vi "basic-intro-log.vi"(0 "Recording Location":string="BI Room 146", 1 "Number of trials":string(combo)="200", 2 "Reward Vol. (uL)":dbl=5.0, 3 "Max number of \nconsecutive trials":string(combo)="3", 4 "Min Licks":i32=1 min=1, 5 "ITI upper (s)":dbl=25.0, 6 "ITI lower (s)":dbl=8.0, 8 "Sequence Directory":path=path "C:/Users/SiapasLab/Desktop/git/wheatley", 9 "Punish Time (s)":dbl=25.0, 10 "Data Saving Directory":path=path "\\\\CA1-17\\ld8007/anesthesia/data", 11 "Trial window (ms)":dbl=3000.0, 12 "Animal Name":string="Mouse", 13 "Trial delay (ms)":dbl=2000.0, 14 "Assay Description":string="Two Choice Audio Discrimination", 15 "Max Time (s)":dbl=3600.0, 16 "Tone Pairs":u16(ring) items=["1: CS+ 10000 Hz, CS- 5000 Hz", "2: CS+ 5800 Hz, CS- 5000 Hz", "3: CS+ 5000 Hz, CS- 10000 Hz", "4: CS+ 8000 Hz, CS- 15000 Hz"], 17 "Protocol":u16(ring)=1 items=["Partial Training 1", "Full Training"]) -> (18 "all rows":i64[](array[numeric]), 20 "Cluster":T2, 21 "Cluster 2":T1)   [LabVIEW 2015]
uses:
  <vilib>/Utility/file.llb/Read Delimited Spreadsheet (I64).vi
panel:
  in  "Ring Refnum":refnum<vi>
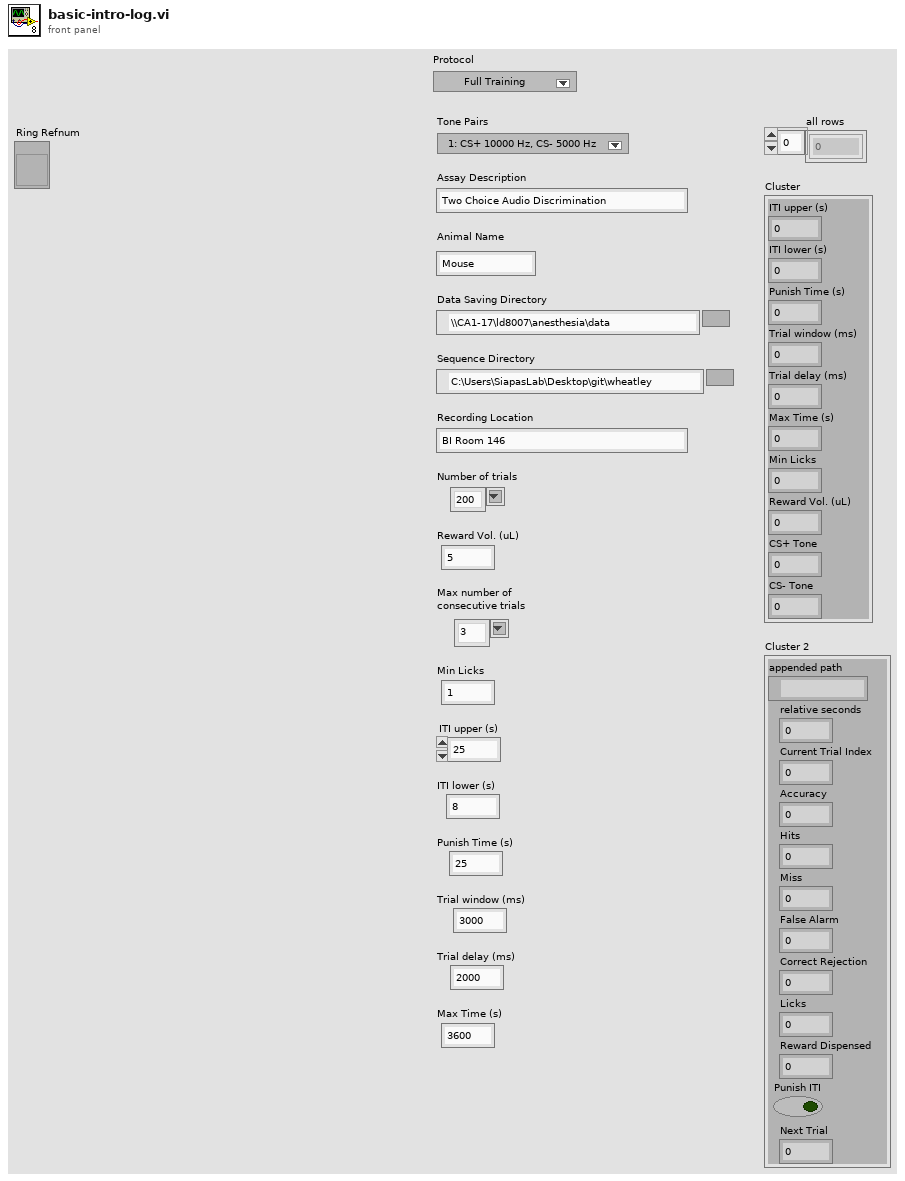
[diagram p1: front panel]
types:
  T1 = cluster{"appended path":path, "relative seconds":dbl, "Current Trial Index":i32, "Accuracy":dbl, "Hits":i32, "Miss":i32, "False Alarm":i32, "Correct Rejection":i32, "Licks":i32, "Reward Dispensed":dbl, "Punish ITI":bool, "Next Trial":i32}
  T2 = cluster{"ITI upper (s)":dbl, "ITI lower (s)":dbl, "Punish Time (s)":dbl, "Trial window (ms)":dbl, "Trial delay (ms)":dbl, "Max Time (s)":dbl, "Min Licks":i32, "Reward Vol. (uL)":dbl, "CS+ Tone":i32, "CS- Tone":i32}
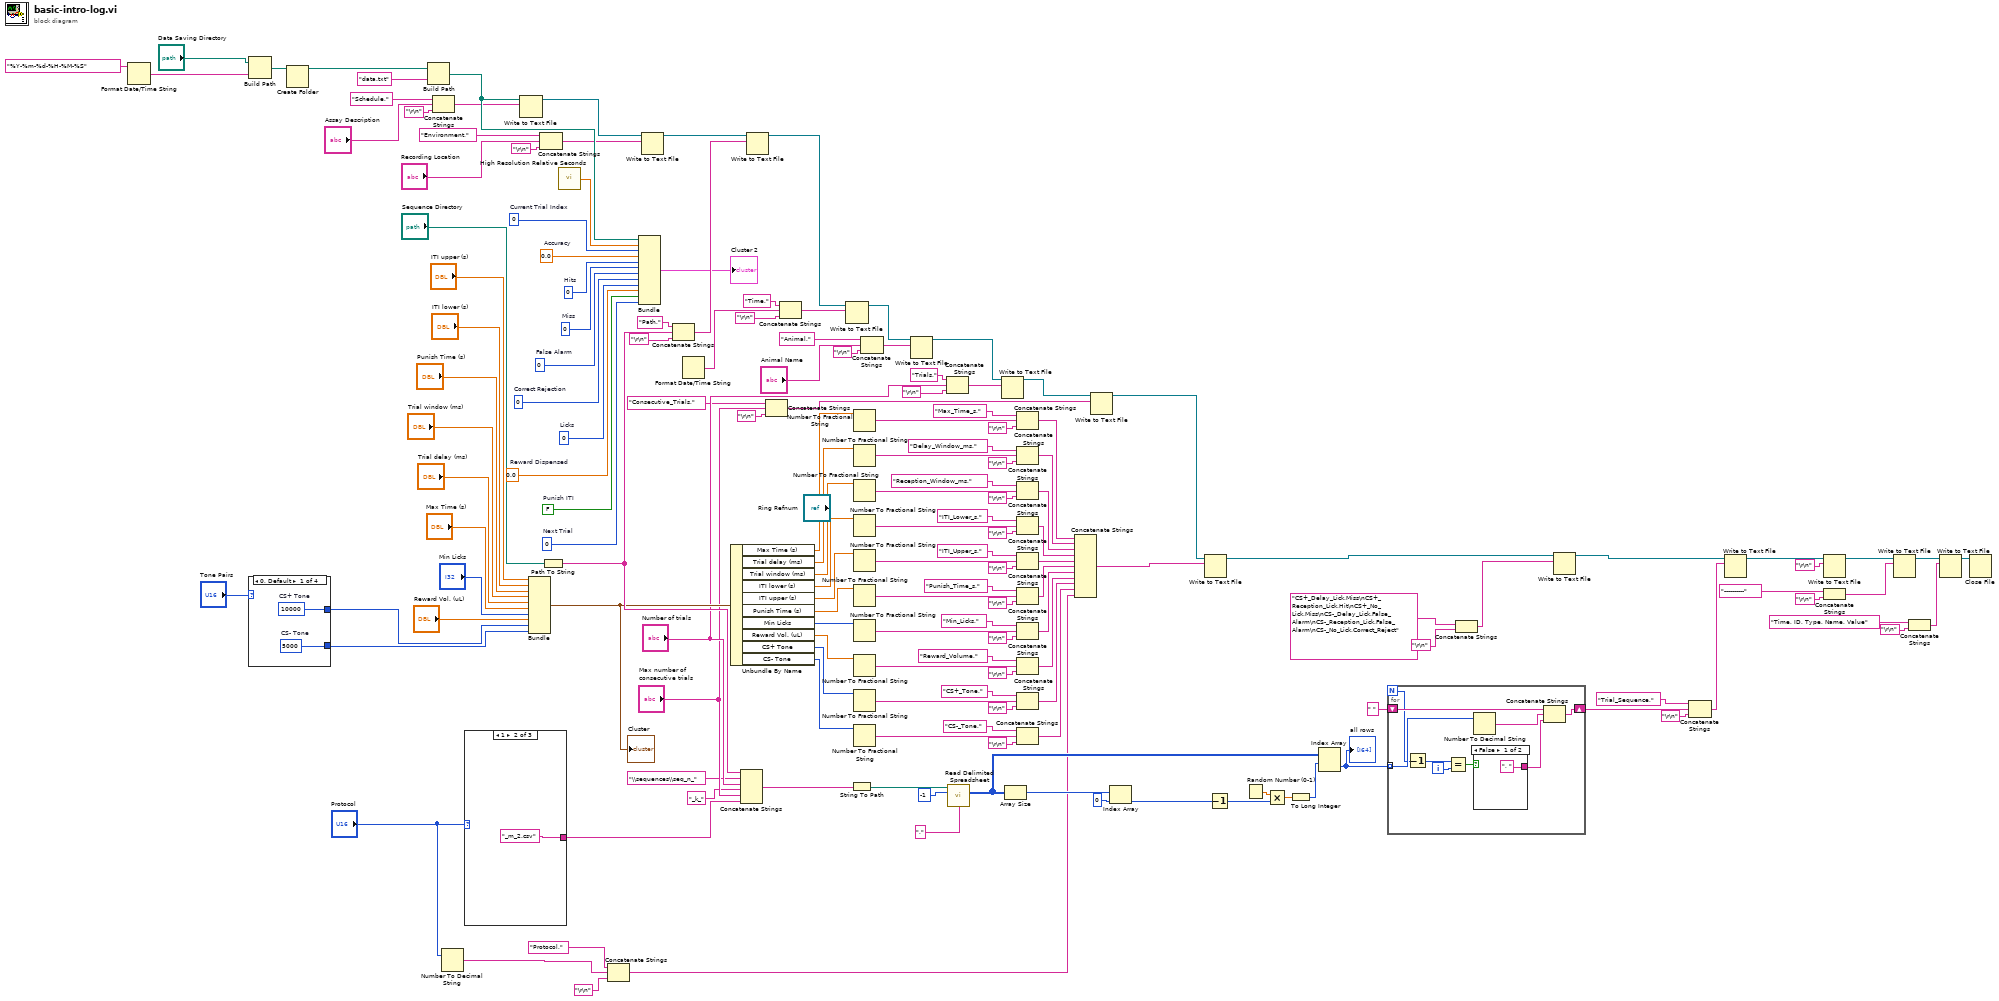
[diagram p0: block diagram]
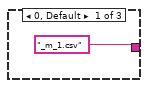
[diagram p2: hidden frame]
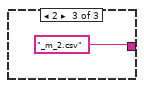
[diagram p3: hidden frame]
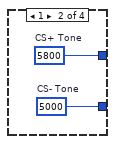
[diagram p4: hidden frame]
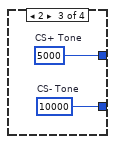
[diagram p5: hidden frame]
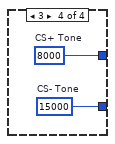
[diagram p6: hidden frame]
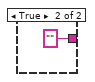
[diagram p7: hidden frame]
diagram:
  w89 = 0  # Next Trial
  w88 = FALSE  # Punish ITI
  w79 = 0.0  # Reward Dispensed
  w78 = 0  # Licks
  w77 = 0  # Correct Rejection
  w76 = 0  # False Alarm
  w73 = 0.0  # Accuracy
  w75 = 0  # Miss
  w74 = 0  # Hits
  w72 = 0  # Current Trial Index
  n1 = Format Date/Time String(time format string (%c)="%Y-%m-%d-%H-%M-%S") -> (date/time string=w157:string)  [unwired: 2 in]
  n2 = Build Path(base path="Data Saving Directory", name or relative path=w157) -> (appended path=w159:path)
  n3 = case shown="0, Default" "Tone Pairs" {
    tunnel: [w162 w163 w165 w167] -> w146
    tunnel: [w161 w164 w166 w168] -> w145
    frame 0, Default {
      w162 = 5000  # CS- Tone
      w161 = 10000  # CS+ Tone
    }
    frame 1 {
      w163 = 5000  # CS- Tone
      w164 = 5800  # CS+ Tone
    }
    frame 2 {
      w165 = 10000  # CS- Tone
      w166 = 5000  # CS+ Tone
    }
    frame 3 {
      w167 = 15000  # CS- Tone
      w168 = 8000  # CS+ Tone
    }
  }
  n4 = Create Folder(path (use dialog)=w159) -> (created path=w160:path)  [unwired: 2 in, 2 out]
  n5 = Build Path(base path=w160, name or relative path="data.txt") -> (appended path=w82:path)
  n6 = Concatenate Strings("Schedule," ("string"), "Assay Description", "\r\n") -> (w26:string)
  n7 = Number To Decimal String(number="Protocol") -> (decimal integer string=w8:string)  [unwired: 1 in]
  n8 = case shown="1" "Protocol" {
    tunnel: ["_m_1.csv" ("string") "_m_2.csv" ("string") "_m_2.csv" ("string")] -> w9
    frame 0, Default {
    }
    frame 1 {
    }
    frame 2 {
    }
  }
  n9 = Write to Text File(file (use dialog)=w82, text=w26) -> (refnum out=w24:refnum<file>)  [unwired: 2 in, 2 out]
  n10 = Bundle("ITI upper (s)"="ITI upper (s)", "ITI lower (s)"="ITI lower (s)", "Punish Time (s)"="Punish Time (s)", "Trial window (ms)"="Trial window (ms)", "Trial delay (ms)"="Trial delay (ms)", "Max Time (s)"="Max Time (s)", "Min Licks"="Min Licks", "Reward Vol. (uL)"="Reward Vol. (uL)", "CS+ Tone"=w145, "CS- Tone"=w146) -> (w92:T2)  [unwired: 1 in]
  "Cluster" <- w92
  n11 = Concatenate Strings("Environment," ("string"), "Recording Location", "\r\n") -> (w30:string)
  n12 = Path To String(path="Sequence Directory") -> (string=w131:string)
  n13 = call <vilib>:"High Resolution Relative Seconds.vi"() -> ("relative seconds"=w70:dbl)
  n14 = Concatenate Strings("Protocol," ("string"), w8, "\r\n") -> (w2:string)
  n15 = Bundle("appended path"=w82, "relative seconds"=w70, "Current Trial Index"=w72, "Accuracy"=w73, "Hits"=w74, "Miss"=w75, "False Alarm"=w76, "Correct Rejection"=w77, "Licks"=w78, "Reward Dispensed"=w79, "Punish ITI"=w88, "Next Trial"=w89) -> (→"Cluster 2":T1)  [unwired: 1 in]
  n16 = Write to Text File(file (use dialog)=w24, text=w30) -> (refnum out=w126:refnum<file>)  [unwired: 2 in, 2 out]
  n17 = Concatenate Strings("Path," ("string"), w131, "\r\n") -> (w128:string)
  n18 = Format Date/Time String() -> (date/time string=w56:string)  [unwired: 3 in]
  n19 = Unbundle By Name(w92) -> ("Max Time (s)"=w93:dbl, "Trial delay (ms)"=w94:dbl, "Trial window (ms)"=w95:dbl, "ITI lower (s)"=w96:dbl, "ITI upper (s)"=w97:dbl, "Punish Time (s)"=w98:dbl, "Min Licks"=w133:i32, "Reward Vol. (uL)"=w141:dbl, "CS+ Tone"=w153:i32, "CS- Tone"=w154:i32)
  n20 = Concatenate Strings(w131, "\\sequences\\seq_n_", "Number of trials", "_k_" ("string"), "Max number of \nconsecutive trials", w9) -> (w17:string)
  n21 = Write to Text File(file (use dialog)=w126, text=w128) -> (refnum out=w127:refnum<file>)  [unwired: 2 in, 2 out]
  n22 = Concatenate Strings("Consecutive_Trials," ("string"), "Max number of \nconsecutive trials", "\r\n") -> (w45:string)
  n23 = Concatenate Strings("Time," ("string"), w56, "\r\n") -> (w34:string)
  n24 = Write to Text File(file (use dialog)=w127, text=w34) -> (refnum out=w35:refnum<file>)  [unwired: 2 in, 2 out]
  n25 = String To Path(string=w17) -> (path=w16:path)
  n26 = Number To Fractional String(number=w93) -> (F-format string=w99:string)  [unwired: 3 in]
  n27 = Number To Fractional String(number=w94) -> (F-format string=w102:string)  [unwired: 3 in]
  n28 = Number To Fractional String(number=w95) -> (F-format string=w105:string)  [unwired: 3 in]
  n29 = Number To Fractional String(number=w96) -> (F-format string=w106:string)  [unwired: 3 in]
  n30 = Number To Fractional String(number=w97) -> (F-format string=w108:string)  [unwired: 3 in]
  n31 = Number To Fractional String(number=w98) -> (F-format string=w111:string)  [unwired: 3 in]
  n32 = Number To Fractional String(number=w133) -> (F-format string=w134:string)  [unwired: 3 in]
  n33 = Number To Fractional String(number=w141) -> (F-format string=w142:string)  [unwired: 3 in]
  n34 = Number To Fractional String(number=w153) -> (F-format string=w152:string)  [unwired: 3 in]
  n35 = Number To Fractional String(number=w154) -> (F-format string=w151:string)  [unwired: 3 in]
  n36 = Concatenate Strings("Animal," ("string"), "Animal Name", "\r\n") -> (w38:string)
  n37 = Write to Text File(file (use dialog)=w35, text=w38) -> (refnum out=w46:refnum<file>)  [unwired: 2 in, 2 out]
  n38 = Concatenate Strings("Trials," ("string"), "Number of trials", "\r\n") -> (w42:string)
  n39 = call-poly <vilib>:"Read Delimited Spreadsheet.vi"("file path (dialog if empty)"=w16, "number of rows (all:-1)"=-1, "delimiter (\\t)"="," ("delimiter (\\t)")) -> ("all rows"=w22:i64[][])  [unwired: 7 in, 5 out]
  n40 = Write to Text File(file (use dialog)=w46, text=w42) -> (refnum out=w47:refnum<file>)  [unwired: 2 in, 2 out]
  n41 = Array Size(array=w22) -> (size(s)=w18:i32[])
  n42 = Concatenate Strings("Max_Time_s," ("string"), w99, "\r\n") -> (w117:string)
  n43 = Concatenate Strings("Delay_Window_ms," ("string"), w102, "\r\n") -> (w118:string)
  n44 = Concatenate Strings("Reception_Window_ms," ("string"), w105, "\r\n") -> (w119:string)
  n45 = Concatenate Strings("ITI_Lower_s," ("string"), w106, "\r\n") -> (w120:string)
  n46 = Concatenate Strings("ITI_Upper_s," ("string"), w108, "\r\n") -> (w121:string)
  n47 = Concatenate Strings("Punish_Time_s," ("string"), w111, "\r\n") -> (w122:string)
  n48 = Concatenate Strings("Min_Licks," ("string"), w134, "\r\n") -> (w137:string)
  n49 = Concatenate Strings("Reward_Volume," ("string"), w142, "\r\n") -> (w143:string)
  n50 = Concatenate Strings("CS+_Tone," ("string"), w152, "\r\n") -> (w155:string)
  n51 = Concatenate Strings("CS-_Tone," ("string"), w151, "\r\n") -> (w156:string)
  n52 = Concatenate Strings(w117, w118, w119, w120, w121, w122, w137, w143, w155, w156, w2) -> (w125:string)
  n53 = Write to Text File(file (use dialog)=w47, text=w45) -> (refnum out=w123:refnum<file>)  [unwired: 2 in, 2 out]
  n54 = Index Array(array=w18, index=0) -> (element=w20:i32)
  n55 = Write to Text File(file (use dialog)=w123, text=w125) -> (refnum out=w124:refnum<file>)  [unwired: 2 in, 2 out]
  n56 = Decrement(x=w20) -> (x-1=w21:i32)
  n57 = Random Number (0-1)() -> (number: 0 to 1=w12:dbl)
  n58 = Multiply(x=w12, y=w21) -> (x*y=w13:dbl)
  n59 = To Long Integer(number=w13) -> (32bit integer=w23:i32)
  n60 = Index Array(array=w22, index (row)=w23) -> (element=w80:i64[])  [unwired: 1 in]
  "all rows" <- w80
  n61 = for {
    N -> [w173]
    shift-right: [w177] -> w90
    shift-left: " " -> [w178]
    tunnel: w80 -> [w180] mode=indexing
    i -> [w176]
    n62 = Decrement(x=w173) -> (x-1=w172:i32)
    n63 = Equal?(x=w172, y=w176) -> (x = y?=w175:bool)
    n64 = Number To Decimal String(number=w180) -> (decimal integer string=w179:string)  [unwired: 1 in]
    n65 = case shown="False" w175 {
      tunnel: [", " ("string") "" ("string")] -> w174
      frame False {
      }
      frame True {
      }
    }
    n66 = Concatenate Strings(w178, w179, w174) -> (w177:string)
  }
  n67 = Concatenate Strings("CS+_Delay_Lick,Miss\nCS+_Reception_Lick,Hit\nCS+_No_Lick,Miss\nCS-_Delay_Lick,False_Alarm\nCS-_Reception_Lick,False_Alarm\nCS-_No_Lick,Correct_Reject", "\r\n") -> (w3:string)
  n68 = Write to Text File(file (use dialog)=w124, text=w3) -> (refnum out=w91:refnum<file>)  [unwired: 2 in, 2 out]
  n69 = Concatenate Strings("Trial_Sequence," ("string"), w90, "\r\n") -> (w59:string)
  n70 = Write to Text File(file (use dialog)=w91, text=w59) -> (refnum out=w58:refnum<file>)  [unwired: 2 in, 2 out]
  n71 = Write to Text File(file (use dialog)=w58, text="\r\n") -> (refnum out=w52:refnum<file>)  [unwired: 2 in, 2 out]
  n72 = Concatenate Strings("----------" ("string"), "\r\n") -> (w53:string)
  n73 = Write to Text File(file (use dialog)=w52, text=w53) -> (refnum out=w85:refnum<file>)  [unwired: 2 in, 2 out]
  n74 = Concatenate Strings("Time, ID, Type, Name, Value" ("string"), "\r\n") -> (w87:string)
  n75 = Write to Text File(file (use dialog)=w85, text=w87) -> (refnum out=w86:refnum<file>)  [unwired: 2 in, 2 out]
  n76 = Close File(refnum=w86) -> ()  [unwired: 1 in, 2 out]
